vi "checkTimeout.vi"(8 "error in (no error)":errorcluster, 10 "ElectrometerController in":refnum<class "ElectrometerController.lvclass">, 11 "SetDurationReading in":refnum<class "SetDurationReading.lvclass">) -> (0 "error out":errorcluster, 1 "timeout?":bool, 2 "ElectrometerController out":refnum<class "ElectrometerController.lvclass">, 3 "SetDurationReading out":refnum<class "SetDurationReading.lvclass">)   [LabVIEW 2016, in "SetDurationReading.lvclass"]
uses:
  SetDurationReading.lvclass
  ElectrometerController/ElectrometerController.lvclass
  Electrometer.lvclass
  ElectrometerConfiguration/ElectrometerInternalConfiguration.lvclass
  State.lvclass
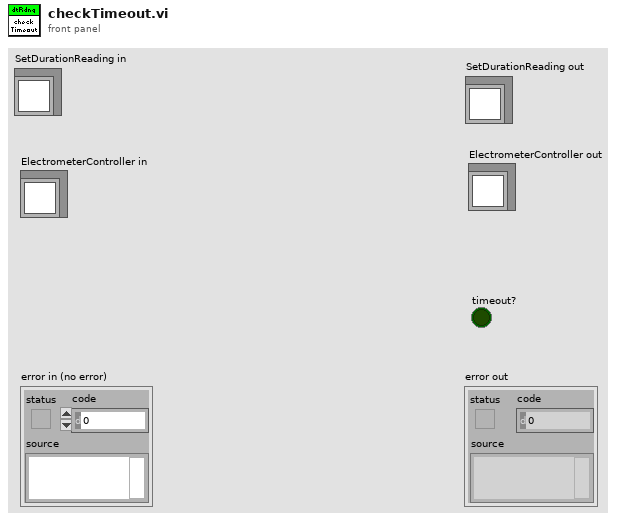
[diagram p1: front panel]
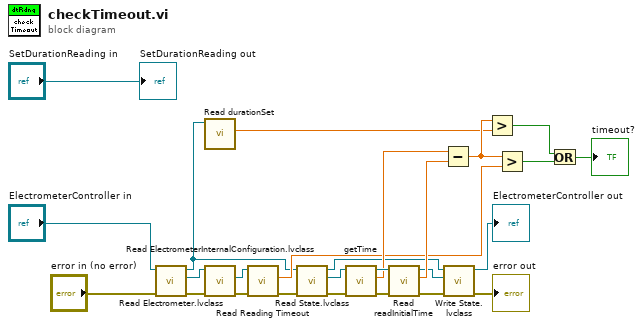
[diagram p0: block diagram]
diagram:
  n1 = call-dynamic "Read Electrometer.lvclass.vi"("error in (no error)"="error in (no error)", "ElectrometerController in"="ElectrometerController in") -> ("error out"=w22:errorcluster, "Electrometer.lvclass"=w25:refnum<class "Electrometer.lvclass">, "ElectrometerController out"=w4:refnum<class "ElectrometerController.lvclass">)  [unwired: 7 in]
  n2 = call-dynamic "Read durationSet.vi"("ElectrometerController in"=w4) -> ("durationSet"=w2:dbl)  [unwired: 8 in, 2 out]
  n3 = call-dynamic "Read ElectrometerInternalConfiguration.lvclass.vi"("error in (no error)"=w22, "Electrometer in"=w25) -> ("error out"=w23:errorcluster, "ElectrometerInternalConfiguration.lvclass"=w24:refnum<class "ElectrometerInternalConfiguration.lvclass">)  [unwired: 7 in, 1 out]
  n4 = call-dynamic "Read Reading Timeout.vi"("error in (no error)"=w23, "ElectrometerInternalConfiguration in"=w24) -> ("error out"=w18:errorcluster, "Reading Timeout"=w12:dbl)  [unwired: 7 in, 1 out]
  n5 = call-dynamic "Read State.lvclass.vi"("error in (no error)"=w18, "ElectrometerController in"=w4) -> ("error out"=w16:errorcluster, "State.lvclass"=w17:refnum<class "State.lvclass">, "ElectrometerController out"=w13:refnum<class "ElectrometerController.lvclass">)  [unwired: 7 in]
  n6 = call-dynamic "getTime.vi"("error in (no error)"=w16, "State in"=w17) -> ("error out"=w21:errorcluster, "relative seconds"=w20:dbl, "State out"=w26:refnum<class "State.lvclass">)  [unwired: 7 in]
  n7 = call-dynamic "Read readInitialTime.vi"("error in (no error)"=w21, "State in"=w26) -> ("error out"=w15:errorcluster, "readInitialTime"=w19:dbl, "State out"=w14:refnum<class "State.lvclass">)  [unwired: 7 in]
  n8 = Subtract(x=w20, y=w19) -> (x-y=w3:dbl)
  n9 = call-dynamic "Write State.lvclass.vi"("error in (no error)"=w15, "State.lvclass"=w14, "ElectrometerController in"=w13) -> ("error out"=→"error out":errorcluster, "ElectrometerController out"=→"ElectrometerController out":refnum<class "ElectrometerController.lvclass">)  [unwired: 7 in]
  n10 = Greater?(x=w3, y=w2) -> (0:w1:bool)
  n11 = Greater?(x=w3, y=w12) -> (0:w6:bool)
  n12 = Or(x=w1, y=w6) -> (x .or. y?=→"timeout?":bool)
  "SetDurationReading out" <- "SetDurationReading in"
